vi "run script line.vi"(8 "error in (no error)":errorcluster caption="에러 입력(에러 없음)", 11 "Script_delay 입력":refnum<class "Script Line_delay.lvclass">) -> (0 "error out":errorcluster caption="에러 출력", 2 "log":string, 3 "Script_delay 출력":refnum<class "Script Line_delay.lvclass">)   [LabVIEW 2020, in "Script Line_delay.lvclass"]
uses:
  Script Line_delay.lvclass
  Script Line_delay.lvclass/Script Line_delay.ctl
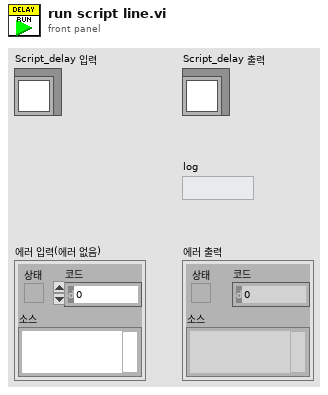
[diagram p1: front panel]
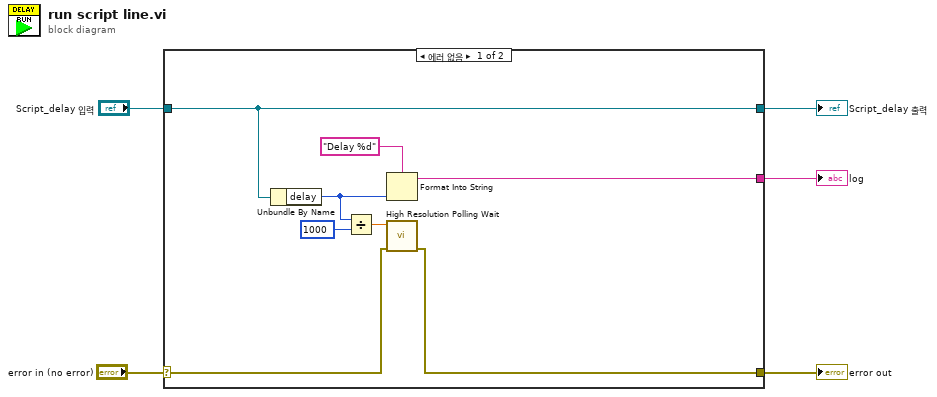
[diagram p0: block diagram]
diagram:
  n1 = case shown="에러 없음" "error in (no error)" {
    selector: "error in (no error)" -> [w7 w15]
    tunnel: [w6 w15] -> w5
    tunnel: [w13 w14] -> w4
    tunnel: "Script_delay 입력" -> [w13 w14]
    tunnel: [w11 _] -> w1
    frame No Error {
      n2 = Unbundle By Name(w13) -> ("delay"=w10:u32)
      n3 = Divide(x=w10, y=u32 1000) -> (x/y=w9:dbl)
      n4 = Format Into String(format string="Delay %d" ("포맷 문자열"), w10) -> (resulting string=w11:string)  [unwired: 2 in, 1 out]
      n5 = call <vilib>:"High Resolution Polling Wait.vi"("error in (no error)"=w7, "seconds to wait"=w9) -> ("error out"=w6:errorcluster)  [unwired: 9 in]
    }
    frame Error {
    }
  }
  "error out" <- w5
  "Script_delay 출력" <- w4
  "log" <- w1
